vi "OrderArrayRobots.vi"(8 "error in (no error)":errorcluster, 11 "Game in":refnum<class "Game.lvclass">) -> (0 "error out":errorcluster, 3 "Game out":refnum<class "Game.lvclass">)   [LabVIEW 2018, in "Game.lvclass"]
uses:
  Game.lvclass
  Utilities_class/Utilities.lvclass
  Robot_class/Robot.lvclass
  Game.lvclass/Game.ctl
  Team_class/Team.lvclass/Team.ctl
  Referee_class/Referee.lvclass/Referee.ctl
  Robot_class/Robot.lvclass/Robot.ctl
  Robot_class/Read id.vi
  Read AllyRef.vi
  Read Referee.vi
  Read Offensive ids.vi
  Read Defensive ids.vi
  Read TestMode.vi
  Read TestMode IDs.vi
  Referee_class/Read our_goalie_id.vi
  Team_class/Read RobotRef.vi
  Team_class/Write RobotRef.vi
  Write AllyRef.vi
  Ally_class/Ally.lvclass
  C:/Users/Ronaldo/Desktop/Phoenix/SSL_AI/Team_class/Team.lvclass
  Referee_class/Referee.lvclass
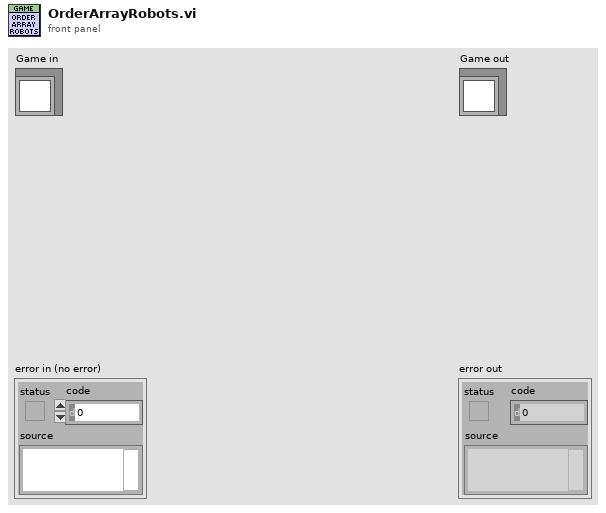
[diagram p1: front panel]
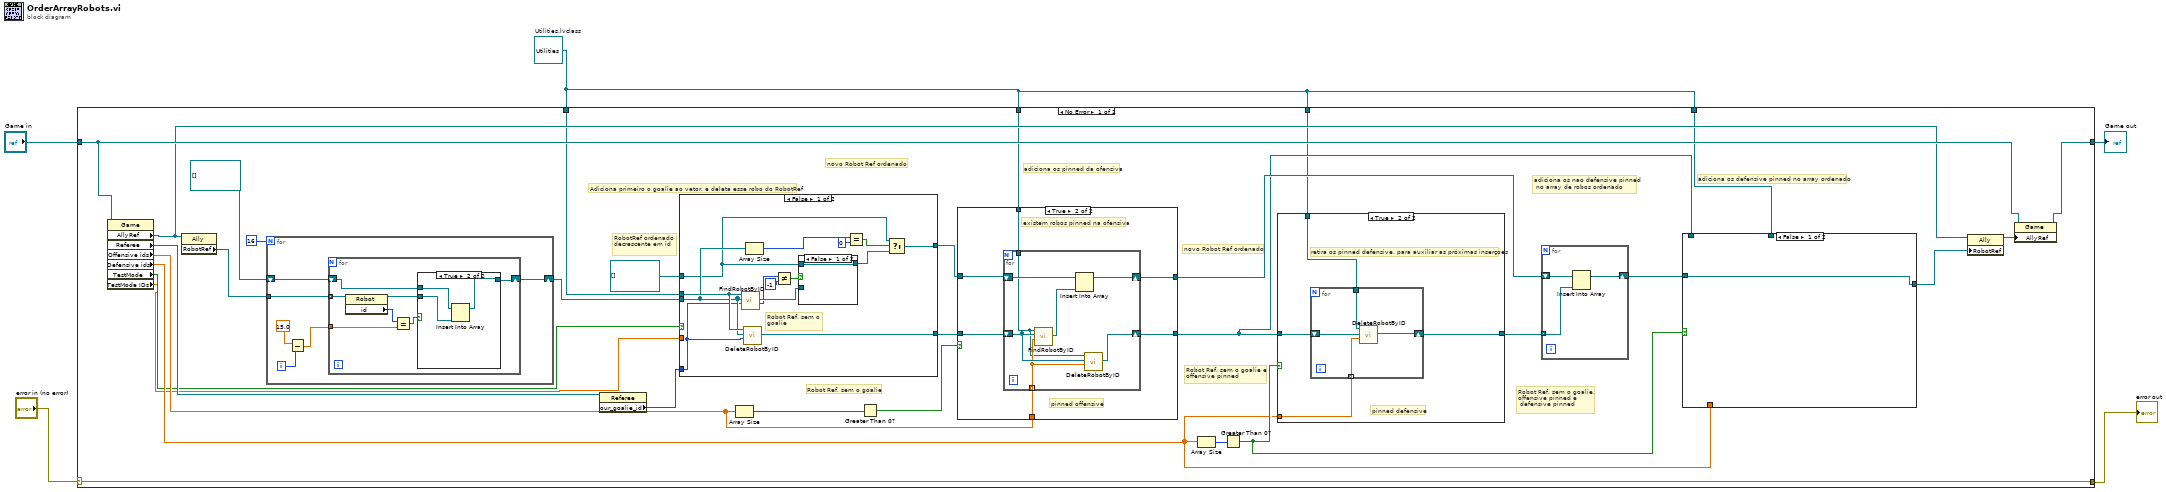
[diagram p0: block diagram]
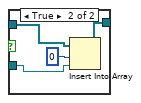
[diagram p2: hidden frame]
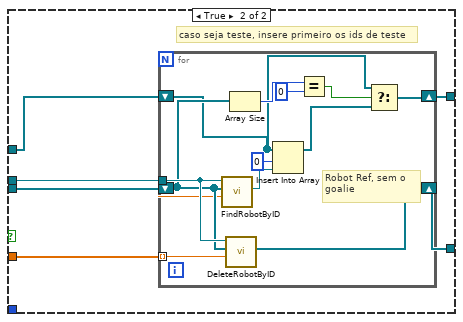
[diagram p3: hidden frame]
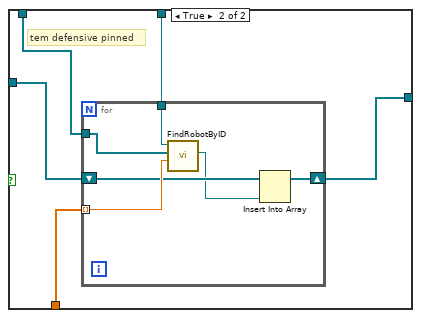
[diagram p7: hidden frame]
diagram:
  w1 = refnum<class "Utilities.lvclass"> refnum  # Utilities.lvclass
  n1 = case shown="No Error" "error in (no error)" {
    selector: "error in (no error)" -> [w36 w131]
    tunnel: [w36 w131] -> w4
    tunnel: [w25 w130] -> w2
    tunnel: "Game in" -> [w26 w130]
    tunnel: w1 -> [w15 _]
    tunnel: w1 -> [w14 _]
    tunnel: w1 -> [w13 _]
    tunnel: w1 -> [w12 _]
    frame No Error {
      # "RobotRef ordenado\ndecrescente em id"
      # "adiciona os defensive pinned no array ordenado"
      # "Robot Ref, sem o goalie, \noffensive pinned e\n defensive pinned"
      # "adiciona os nao defensive pinned\n no array de robos ordenado"
      # "adiciona os pinned da ofensiva"
      # "novo Robot Ref ordenado"
      # "novo Robot Ref ordenado"
      # "Robot Ref, sem o goalie e \noffensive pinned"
      # "Robot Ref, sem o goalie"
      # "Adiciona primeiro o goalie ao vetor, e deleta esse robo do RobotRef"
      n2 = property class="Game"(reference=w26) -> ("AllyRef"=w24:refnum<class "Ally.lvclass">, "Referee"=w35:refnum<class "Referee.lvclass">, "Offensive ids"=w16:dbl[], "Defensive ids"=w19:dbl[], "TestMode"=w7:bool, "TestMode IDs"=w6:dbl[])  [unwired: 1 in, 2 out]
      n3 = property class="Ally"(reference=w24) -> ("RobotRef"=w22:refnum<class "Robot.lvclass">[])  [unwired: 1 in, 2 out]
      n4 = for {
        N: 16 -> [_]
        tunnel: w22 -> [w76]
        shift-right: [w75] -> w11
        shift-left: refnum<class "Robot.lvclass">[] [] -> [w74]
        i -> [w79]
        n5 = Subtract(x=15.0, y=w79) -> (x-y=w77:dbl)
        n6 = for {
          tunnel: w77 -> [w84]
          tunnel: w76 -> [w86] mode=indexing
          shift-right: [w80] -> w75
          shift-left: w74 -> [w81]
          n7 = property class="Robot"(reference=w86) -> (reference out=w82:refnum<class "Robot.lvclass">, "id"=w85:i32)  [unwired: 1 in, 1 out]
          n8 = Equal?(x=w85, y=w84) -> (x = y?=w83:bool)
          n9 = case shown="True" w83 {
            tunnel: w82 -> [_ w90]
            tunnel: [w87 w89] -> w80
            tunnel: w81 -> [w87 w88]
            frame False {
            }
            frame True {
              n10 = Insert Into Array(array=w88, new element=w90) -> (w89:refnum<class "Robot.lvclass">[])  [unwired: 1 in]
            }
          }
        }
      }
      n11 = property class="Referee"(reference=w35) -> ("our_goalie_id"=w8:i32)  [unwired: 1 in, 2 out]
      n12 = case shown="False" w7 {
        tunnel: [w49 w61] -> w20
        tunnel: w15 -> [w48 w60]
        tunnel: w11 -> [w44 w59]
        tunnel: [w43 w58] -> w10
        tunnel: refnum<class "Robot.lvclass">[] [] -> [w40 w57]
        tunnel: w8 -> [w41 _]
        tunnel: w6 -> [_ w56]
        frame False {
          # "Robot Ref, sem o goalie"
          n13 = call-dynamic "FindRobotByID.vi"("id"=w41, "RobotRef"=w44, "Utilities in"=w48) -> ("index"=w38:i32, "Robot"=w50:refnum<class "Robot.lvclass">)  [unwired: 5 in, 2 out]
          n14 = call-dynamic "DeleteRobotByID.vi"("id"=w41, "RobotRef"=w44, "Utilities in"=w48) -> ("RobotRef out"=w49:refnum<class "Robot.lvclass">[])  [unwired: 6 in, 2 out]
          n15 = Array Size(array=w44) -> (size(s)=w47:i32)
          n16 = Not Equal?(x=w38, y=-1) -> (x != y?=w39:bool)
          n17 = case shown="False" w39 {
            tunnel: w50 -> [_ w55]
            tunnel: [w51 w53] -> w42
            tunnel: w40 -> [w51 w52]
            frame False {
            }
            frame True {
              n18 = Insert Into Array(array=w52, index=0, new element=w55) -> (w53:refnum<class "Robot.lvclass">[])
            }
          }
          n19 = Equal?(x=w47, y=0) -> (x = y?=w45:bool)
          n20 = Select(t=w40, s=w45, f=w42) -> (s? t:f=w43:refnum<class "Robot.lvclass">[])
        }
        frame True {
          # "caso seja teste, insere primeiro os ids de teste"
          n21 = for {
            tunnel: w60 -> [w70]
            tunnel: w56 -> [w63] mode=indexing
            shift-right: [w71] -> w61
            shift-left: w59 -> [w66]
            shift-right: [w65] -> w58
            shift-left: w57 -> [w62]
            # "Robot Ref, sem o goalie"
            n22 = call-dynamic "FindRobotByID.vi"("id"=w63, "RobotRef"=w66, "Utilities in"=w70) -> ("Robot"=w73:refnum<class "Robot.lvclass">)  [unwired: 5 in, 3 out]
            n23 = call-dynamic "DeleteRobotByID.vi"("id"=w63, "RobotRef"=w66, "Utilities in"=w70) -> ("RobotRef out"=w71:refnum<class "Robot.lvclass">[])  [unwired: 6 in, 2 out]
            n24 = Array Size(array=w66) -> (size(s)=w69:i32)
            n25 = Insert Into Array(array=w62, index=0, new element=w73) -> (w64:refnum<class "Robot.lvclass">[])
            n26 = Equal?(x=w69, y=0) -> (x = y?=w67:bool)
            n27 = Select(t=w62, s=w67, f=w64) -> (s? t:f=w65:refnum<class "Robot.lvclass">[])
          }
        }
      }
      n28 = Array Size(array=w16) -> (size(s)=w34:i32)
      n29 = Greater Than 0?(x=w34) -> (x > 0?=w33:bool)
      n30 = case shown="True" w33 {
        tunnel: w10 -> [w92 w98]
        tunnel: w20 -> [w91 w97]
        tunnel: [w92 w96] -> w18
        tunnel: [w91 w95] -> w17
        tunnel: w16 -> [_ w94]
        tunnel: w14 -> [_ w93]
        frame False {
          # "nao tem robos pinned, entao nao adiciona nada ao array"
        }
        frame True {
          # "pinned offensive"
          # "existem robos pinned na ofensiva"
          n31 = for {
            shift-right: [w100] -> w95
            shift-left: w97 -> [w102]
            shift-right: [w104] -> w96
            shift-left: w98 -> [w105]
            tunnel: w94 -> [w101] mode=indexing
            tunnel: w93 -> [w99]
            n32 = call-dynamic "FindRobotByID.vi"("id"=w101, "RobotRef"=w102, "Utilities in"=w99) -> ("Robot"=w103:refnum<class "Robot.lvclass">)  [unwired: 5 in, 3 out]
            n33 = Insert Into Array(array=w105, new element=w103) -> (w104:refnum<class "Robot.lvclass">[])  [unwired: 1 in]
            n34 = call-dynamic "DeleteRobotByID.vi"("id"=w101, "RobotRef"=w102, "Utilities in"=w99) -> ("RobotRef out"=w100:refnum<class "Robot.lvclass">[])  [unwired: 6 in, 2 out]
          }
        }
      }
      n35 = Array Size(array=w19) -> (size(s)=w31:i32)
      n36 = Greater Than 0?(x=w31) -> (x > 0?=w30:bool)
      n37 = case shown="True" w30 {
        tunnel: w17 -> [w106 w110]
        tunnel: w19 -> [_ w109]
        tunnel: [w106 w108] -> w32
        tunnel: w13 -> [_ w107]
        frame False {
        }
        frame True {
          # "retira os pinned defensive, para auxiliar as próximas inserçoes"
          # "pinned defensive"
          n38 = for {
            shift-right: [w113] -> w108
            shift-left: w110 -> [w114]
            tunnel: w109 -> [w112] mode=indexing
            tunnel: w107 -> [w111]
            n39 = call-dynamic "DeleteRobotByID.vi"("id"=w112, "RobotRef"=w114, "Utilities in"=w111) -> ("RobotRef out"=w113:refnum<class "Robot.lvclass">[])  [unwired: 6 in, 2 out]
          }
        }
      }
      n40 = for {
        shift-right: [w127] -> w29
        shift-left: w18 -> [w129]
        tunnel: w32 -> [w128] mode=indexing
        n41 = Insert Into Array(array=w129, new element=w128) -> (w127:refnum<class "Robot.lvclass">[])  [unwired: 1 in]
      }
      n42 = case shown="False" w30 {
        tunnel: w29 -> [w115 w120]
        tunnel: [w115 w119] -> w28
        tunnel: w19 -> [_ w118]
        tunnel: w17 -> [_ w117]
        tunnel: w12 -> [_ w116]
        frame False {
        }
        frame True {
          # "tem defensive pinned"
          n43 = for {
            shift-right: [w122] -> w119
            shift-left: w120 -> [w124]
            tunnel: w118 -> [w125] mode=indexing
            tunnel: w117 -> [w126]
            tunnel: w116 -> [w121]
            n44 = call-dynamic "FindRobotByID.vi"("id"=w125, "RobotRef"=w126, "Utilities in"=w121) -> ("Robot"=w123:refnum<class "Robot.lvclass">)  [unwired: 5 in, 3 out]
            n45 = Insert Into Array(array=w124, new element=w123) -> (w122:refnum<class "Robot.lvclass">[])  [unwired: 1 in]
          }
        }
      }
      n46 = property class="Ally"(reference=w24, "RobotRef"=w28) -> (reference out=w27:refnum<class "Ally.lvclass">)  [unwired: 1 in, 1 out]
      n47 = property class="Game"(reference=w26, "AllyRef"=w27) -> (reference out=w25:refnum<class "Game.lvclass">)  [unwired: 1 in, 1 out]
    }
    frame Error {
    }
  }
  "error out" <- w4
  "Game out" <- w2
